vi "Build Channel Cluster Array.vi"(11 "Channels Amount":u8) -> (3 "Channels out":cluster{"Channels":T1[]})   [LabVIEW 2023, in "Chiller Cluster.lvclass"]
uses:
  Chiller Cluster.lvclass
  Utilities/Utilities.lvlib
  Utilities/Channel.ctl
panel:
  in  "Chiller Cluster.lvclass":refnum<class "Chiller Cluster.lvclass">
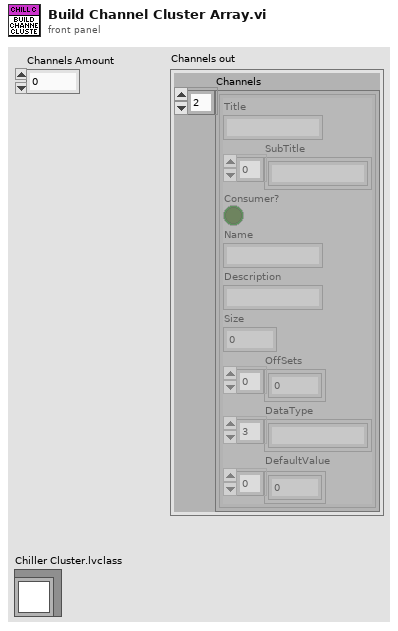
[diagram p1: front panel]
types:
  T1 = typedef "Utilities.lvlib/Channel.ctl" = cluster{"Title":string, "SubTitle":string[], "Consumer?":bool, "Name":string, "Description":string, "Size":i32, "OffSets":i32[], "DataType":string[], "DefaultValue":dbl[]}
  T2 = cluster{"OnOff.ACT":bool, "ErrorAcknowledge.ACT":bool}
  T3 = cluster{"OnOff.STS":i32, "Error.STS":i32, "Watchdog.STS":i32}
  T4 = cluster{"ErrorAcknowledge.ACT":bool, "OutputEnable.ACT":bool, "ControlMode.CTL":u16, "Temperature.SP":dbl, "TemperatureMIN.SP":dbl, "TemperatureMAX.SP":dbl, "TemperatureGrad.SP":dbl, "Pressure.SP":dbl, "PressureMIN.SP":dbl, "PressureMAX.SP":dbl, "PressureGrad.SP":dbl, "Flow.SP":dbl, "FlowMIN.SP":dbl, "FlowMAX.SP":dbl, "FlowGrad.SP":dbl}[]
  T5 = cluster{"Error.STS":i32, "OutputEnable.STS":i32, "ControlMode.STS":u16, "Temperature.AV":dbl, "Pressure.AV":dbl, "Flow.AV":dbl}[]
  T6 = cluster{"Error.STS":i32, "OutputEnable.STS":i32, "ControlMode.STS":u16, "Temperature.AV":dbl, "Pressure.AV":dbl, "Flow.AV":dbl}
  T7 = cluster{"ErrorAcknowledge.ACT":bool, "OutputEnable.ACT":bool, "ControlMode.CTL":u16, "Temperature.SP":dbl, "TemperatureMIN.SP":dbl, "TemperatureMAX.SP":dbl, "TemperatureGrad.SP":dbl, "Pressure.SP":dbl, "PressureMIN.SP":dbl, "PressureMAX.SP":dbl, "PressureGrad.SP":dbl, "Flow.SP":dbl, "FlowMIN.SP":dbl, "FlowMAX.SP":dbl, "FlowGrad.SP":dbl}
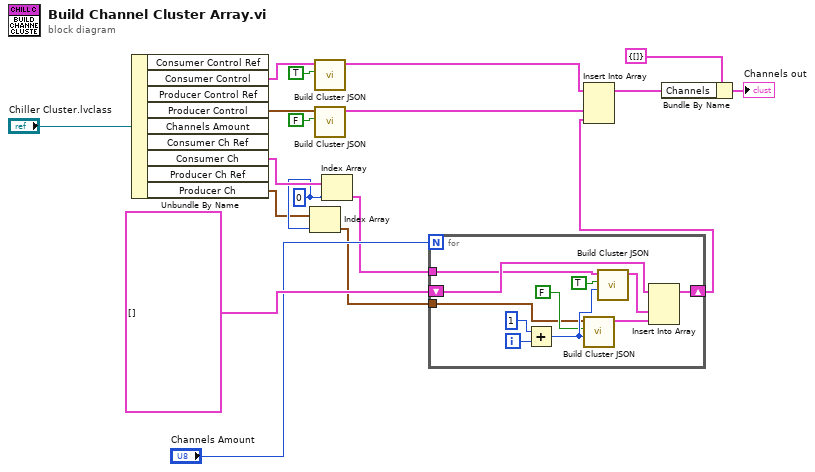
[diagram p0: block diagram]
diagram:
  w3 = 0 ("index")
  n1 = Unbundle By Name("Chiller Cluster.lvclass") -> ("Consumer Control"=w8:T2, "Producer Control"=w7:T3, "Consumer Ch"=w5:T4, "Producer Ch"=w2:T5)  [unwired: 5 out]
  n2 = Index Array(array=w2, index=w3) -> (element=w1:T6)
  n3 = call "Build Cluster JSON.vi"("Consumer?"=TRUE, "Cluster"=w8) -> ("Array"=w15:T1[])  [unwired: 9 in]
  n4 = call "Build Cluster JSON.vi"("Consumer?"=FALSE, "Cluster"=w7) -> ("Array"=w14:T1[])  [unwired: 9 in]
  n5 = Index Array(array=w5, index=w3) -> (element=w4:T7)
  n6 = for {
    N: "Channels Amount" -> [_]
    shift-right: [w25] -> w12
    shift-left: T1[] [] -> [w26]
    tunnel: w4 -> [w21]
    tunnel: w1 -> [w19]
    i -> [w24]
    n7 = Add(x=1, y=w24) -> (x+y=w22:i32)
    n8 = call "Build Cluster JSON.vi"("Channels Amount"=w22, "Consumer?"=FALSE, "Cluster"=w19) -> ("Array"=w27:T1[])  [unwired: 8 in]
    n9 = call "Build Cluster JSON.vi"("Channels Amount"=w22, "Consumer?"=TRUE, "Cluster"=w21) -> ("Array"=w28:T1[])  [unwired: 8 in]
    n10 = Insert Into Array(array=w26, new element #1=w28, new element #2=w27) -> (w25:T1[])  [unwired: 1 in]
  }
  n11 = Insert Into Array(array=w15, new element #1=w14, new element #2=w12) -> (w10:T1[])  [unwired: 1 in]
  n12 = Bundle By Name(cluster=cluster{"Channels":T1[]} {"Channels"=[]} ("Channels in"), "Channels"=w10) -> (→"Channels out":cluster{"Channels":T1[]})
